vi "Revision Query.vi"(8 "error in (no error)":errorcluster, 11 "VISA resource name":refnum<visa-resource-name>) -> (0 "error out":errorcluster, 2 "Instrument Driver Revision":string, 3 "VISA resource name out":refnum<visa-resource-name>)   [LabVIEW 2020, in "Anritsu Signal Analyzer Series.lvlib"]
doc: "Queries the current instrument firmware revision and instrument driver revision.\n\nRefer to the Readme file for detailed driver information including modification history."
uses:
  Anritsu Signal Analyzer Series.lvlib
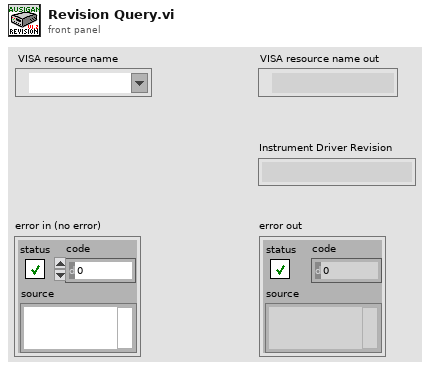
[diagram p1: front panel]
types:
  T1 = cluster{"Major":u16, "Minor":u16, "Fix":u16, "Build":u16}
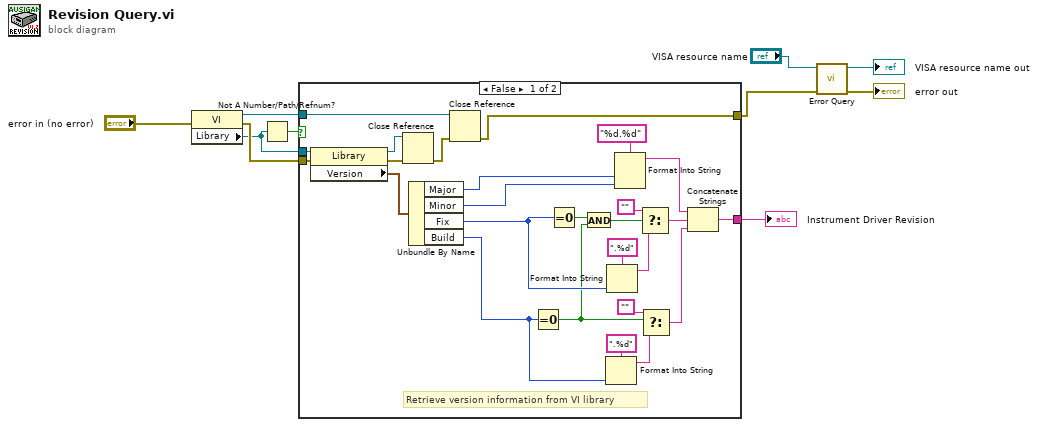
[diagram p0: block diagram]
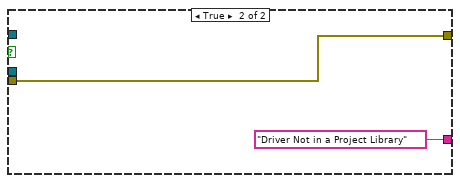
[diagram p2: hidden frame]
diagram:
  n1 = property class="VI"(error in="error in (no error)") -> (reference out=w6:refnum<vi>, error out=w5:errorcluster, "Library"=w4:refnum<vi>)  [unwired: 1 in]
  n2 = Not A Number/Path/Refnum?(number/path/refnum=w4) -> (NaN/Path/Refnum?=w3:bool)
  n3 = case shown="False" w3 {
    tunnel: w6 -> [w33 _]
    tunnel: w5 -> [w18 w38]
    tunnel: [w13 w38] -> w2
    tunnel: [w12 "Driver Not in a Project Library"] -> w8
    tunnel: w4 -> [w11 _]
    frame False {
      # "Retrieve version information from VI library"
      n4 = property class="Library"(reference=w11, error in=w18) -> (reference out=w35:refnum<vi>, error out=w36:errorcluster, "Version"=w32:T1)
      n5 = Close Reference(reference=w35, error in (no error)=w36) -> (error out=w34:errorcluster)
      n6 = Unbundle By Name(w32) -> ("Major"=w21:u16, "Minor"=w20:u16, "Fix"=w17:u16, "Build"=w19:u16)
      n7 = Close Reference(reference=w33, error in (no error)=w34) -> (error out=w13:errorcluster)
      n8 = Equal To 0?(x=w19) -> (x = 0?=w15:bool)
      n9 = Equal To 0?(x=w17) -> (x = 0?=w16:bool)
      n10 = And(x=w16, y=w15) -> (x .and. y?=w14:bool)
      n11 = Format Into String(format string=".%d", w19) -> (resulting string=w25:string)  [unwired: 2 in, 1 out]
      n12 = Format Into String(format string=".%d", w17) -> (resulting string=w29:string)  [unwired: 2 in, 1 out]
      n13 = Format Into String(format string="%d.%d", w21, w20) -> (resulting string=w27:string)  [unwired: 2 in, 1 out]
      n14 = Select(t="", s=w14, f=w29) -> (s? t:f=w26:string)
      n15 = Select(t="", s=w15, f=w25) -> (s? t:f=w22:string)
      n16 = Concatenate Strings(w27, w26, w22) -> (w12:string)
    }
    frame True {
    }
  }
  "Instrument Driver Revision" <- w8
  n17 = call "Error Query.vi"("error in (no error)"=w2, "VISA resource name"="VISA resource name") -> ("error out"=→"error out":errorcluster, "VISA resource name out"=→"VISA resource name out":refnum<visa-resource-name>)  [unwired: 6 in, 2 out]
